vi "Get Color Scale Information.vi"(8 "Error In":errorcluster, 11 "ColorRamp in":refnum<vi>) -> (0 "Error Out":errorcluster, 3 "Image Color Scale Information":T1)   [LabVIEW 2021, in "Palette.lvlib"]
uses:
  Palette.lvlib
  Image/Image Color Scale Information.ctl
  Image/Image.lvlib
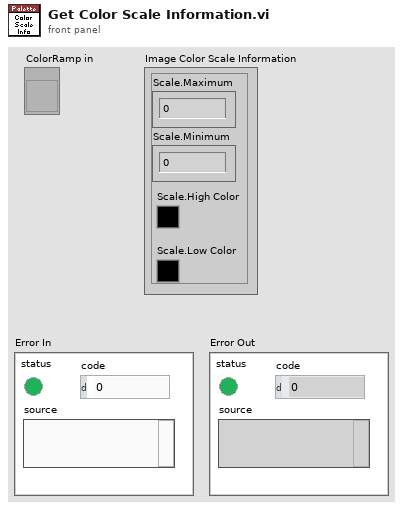
[diagram p1: front panel]
types:
  T1 = typedef "Image.lvlib/Image Color Scale Information.ctl" = cluster{"Scale.Maximum":dbl, "Scale.Minimum":dbl, "Scale.High Color":u32, "Scale.Low Color":u32}
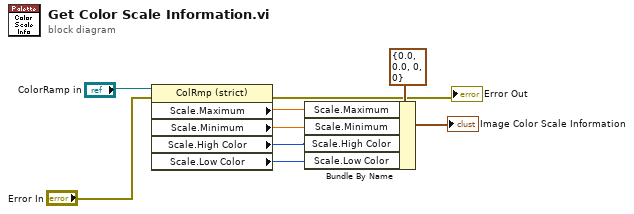
[diagram p0: block diagram]
diagram:
  n1 = property class="ColRmp (strict)"(reference="ColorRamp in", error in="Error In") -> (error out=→"Error Out":errorcluster, "Scale.Maximum"=w6:dbl, "Scale.Minimum"=w5:dbl, "Scale.High Color"=w4:u32, "Scale.Low Color"=w3:u32)  [unwired: 1 out]
  n2 = Bundle By Name(cluster=T1 {"Scale.Maximum"=0.0, "Scale.Minimum"=0.0, "Scale.High Color"=0, "Scale.Low Color"=0} ("Image Color Scale Information"), "Scale.Maximum"=w6, "Scale.Minimum"=w5, "Scale.High Color"=w4, "Scale.Low Color"=w3) -> (→"Image Color Scale Information":T1)
